vi "DriveModuleControl_TravTunePID.vi"(8 "error in":errorcluster, 9 "Actual State":T1={"Speed"=0.0, "Angle"={"VALUE"=0.0, "COS"=1.0, "SIN"=0.0}} {"Angle"."SIN" format="%13.4f"; "Angle"."COS" format="%13.4f"; "Angle"."VALUE" format="%13.4f"}, 10 "Desired State":T1={"Speed"=0.0, "Angle"={"VALUE"=0.0, "COS"=1.0, "SIN"=0.0}} {"Angle"."SIN" format="%13.4f"; "Angle"."COS" format="%13.4f"; "Angle"."VALUE" format="%13.4f"}, 11 "ModualNamePrefix":i32) -> (0 "error out":errorcluster)   [LabVIEW 2023]
uses:
  <vilib>/Rock Robotics/WPI/ThirdParty/JAS_Junk/TrajLib/TypeDef/SWERVE_DRIVE_MODULE_STATE.ctl
  <vilib>/Rock Robotics/WPI/ThirdParty/JAS_Junk/TrajLib/TypeDef/ROTATION2D.ctl
  <vilib>/Rock Robotics/WPI/ThirdParty/REV Robotics/REVLib/Typedef/Spark MAX Control Type.ctl
  <vilib>/Rock Robotics/WPI/ThirdParty/JAS_Junk/TrajLib/Rotation2d_Minus.vi
  <vilib>/Rock Robotics/WPI/ThirdParty/JAS_Junk/TrajLib/Rotation2d_GetRadians.vi
  <vilib>/Rock Robotics/WPI/ThirdParty/JAS_Junk/TrajLib/SwerveModuleState_New.vi
  <vilib>/Rock Robotics/WPI/ThirdParty/JAS_Junk/TrajLib/Rotation2d_RotateBy.vi
  <vilib>/Rock Robotics/WPI/ThirdParty/JAS_Junk/TrajLib/Rotation2d_CreateAngle.vi
  <vilib>/Rock Robotics/WPI/ThirdParty/JAS_Junk/TrajLib/SimpleMotorFF_Calculate.vi
  <vilib>/Rock Robotics/WPI/ThirdParty/JAS_Junk/TrajLib/PIDController_AtSetpoint.vi
  <vilib>/Rock Robotics/WPI/ThirdParty/JAS_Junk/TrajLib/PIDController_SetPIDF.vi
  <vilib>/Rock Robotics/WPI/ThirdParty/JAS_Junk/TrajLib/PIDController_SetDerivativeFilter.vi
  <vilib>/Rock Robotics/WPI/ThirdParty/JAS_Junk/TrajLib/PIDController_SetIntegratorRange.vi
  <vilib>/Rock Robotics/WPI/ThirdParty/JAS_Junk/TrajLib/PIDController_SetTolerancePandV.vi
  <vilib>/Rock Robotics/WPI/ThirdParty/JAS_Junk/TrajLib/PIDController_DisableContinousInput.vi
  <vilib>/Rock Robotics/WPI/ThirdParty/JAS_Junk/TrajLib/PIDController_EnableContinousInput.vi
  <vilib>/Rock Robotics/WPI/ThirdParty/JAS_Junk/TrajLib/PIDController_Reset.vi
  <vilib>/Rock Robotics/WPI/ThirdParty/JAS_Junk/TrajLib/PIDController_New.vi
  <vilib>/Rock Robotics/WPI/ThirdParty/JAS_Junk/TrajLib/PIDController_SetOutputLimits.vi
  <vilib>/Rock Robotics/WPI/ThirdParty/JAS_Junk/TrajLib/VI/PIDController_SetIntegratorZone.vi
  <vilib>/Rock Robotics/WPI/ThirdParty/JAS_Junk/TrajLib/Timer_New.vi
  <vilib>/Rock Robotics/WPI/ThirdParty/JAS_Junk/TrajLib/Rotation2d_UnaryMinus.vi
  <vilib>/Rock Robotics/WPI/ThirdParty/JAS_Junk/TrajLib/Rotation2d_CreateXY.vi
  <vilib>/Rock Robotics/WPI/ThirdParty/JAS_Junk/TrajLib/PIDController_NewPeriod.vi
  <vilib>/Rock Robotics/WPI/ThirdParty/JAS_Junk/TrajLib/Util_CalcDist.vi
  <vilib>/Rock Robotics/SystemInterfaces/NetworkCommunication/NetComm_UsageReport_report.vi
  DriveGlobal.vi
  <vilib>/Utility/semaphor.llb/Obtain Semaphore Reference.vi
  <vilib>/Rock Robotics/WPI/ThirdParty/JAS_Junk/TrajLib/Timer_Reset.vi
  <vilib>/Rock Robotics/WPI/ThirdParty/JAS_Junk/TrajLib/Timer_Start.vi
  <vilib>/Rock Robotics/WPI/ThirdParty/JAS_Junk/TrajLib/Timer_Stop.vi
  <vilib>/Rock Robotics/WPI/ThirdParty/JAS_Junk/TrajLib/Timer_HasPeriodPassedOnce.vi
  <vilib>/Rock Robotics/WPI/ThirdParty/Phoenix6/Phoenix6_Device_RefNumRegistryGet.vi
  <vilib>/Rock Robotics/WPI/MotorControl/WPI_MotorControlRefNum Registry Get.vi
  <vilib>/Rock Robotics/WPI/ThirdParty/JAS_Junk/TrajLib/Globals/Util_LibraryGlobals.vi
  <vilib>/Rock Robotics/WPI/ThirdParty/JAS_Junk/TrajLib/PIDController_AdvCalculate_FF_Sp_Pv.vi
  DriveTuningGlobals.vi
  <vilib>/Rock Robotics/WPI/ThirdParty/JAS_Junk/TrajLib/Trajectory_Library.lvlib
panel:
  out "TravelMotorDmd":dbl
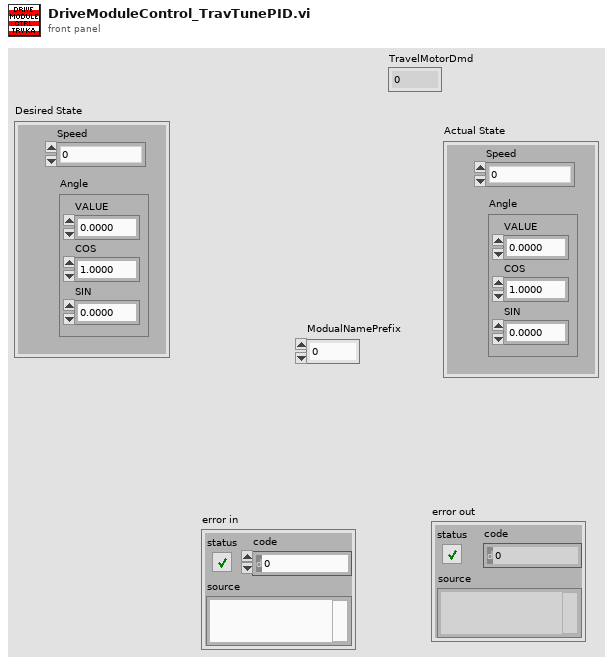
[diagram p1: front panel]
types:
  T1 = typedef "Trajectory_Library.lvlib/SWERVE_DRIVE_MODULE_STATE.ctl" = cluster{"Speed":dbl, "Angle":T2}
  T2 = typedef "Trajectory_Library.lvlib/ROTATION2D.ctl" = cluster{"VALUE":dbl, "COS":dbl, "SIN":dbl}
  T3 = typedef "Spark MAX Control Type.ctl" = enum16{"Percent VBus", "Voltage", "Velocity", "Position", "Smart Motion", "Current", "Smart Velocity", "MAXMotion Position", "MAXMotion Velocity"}
  T4 = enum16{"Ziegler Nicols - Fast", "Ziegler Nicols - Normal", "Ziegler Nicols - Slow", "CHR regulator - 0% overshoot", "CHR regulator - 20% overshoot", "CHR servo - 0 % overshoot", "CHR servo - 20% overshoot"}
  T5 = typedef "WPI_MotorControlDeviceRef.ctl" = cluster{"DeviceStatus":errorcluster, "Type":T6, "PWM":cluster{"PWM Channel":T7, "DeadBand":T8}, "CAN":cluster{"Device Number":u8, "SetOutput VI Ref":variant, "GetOutput VI Ref":variant, "Enable VI Ref":variant, "Disable VI Ref":variant, "Data":variant}, "Invert":bool, "DIO PWM":cluster{"PWM \"Enable\" Channel":T7, "DIOChannel":T9, "PWM Rate":dbl}}
  T6 = typedef "WPI_MotorControlType.ctl" = enum16{"PWM", "CAN", "DIO PWM"}
  T7 = typedef "FPGA_DIOPWMChannel.ctl" = enum8{"PWM 0", "PWM 1", "PWM 2", "PWM 3", "PWM 4", "PWM 5", "PWM 6", "PWM 7", "PWM 8", "PWM 9", "PWM MXP 0", "PWM MXP 1", "PWM MXP 2", "PWM MXP 3", "PWM MXP 4", "PWM MXP 5", "PWM MXP 6", "PWM MXP 7", "PWM MXP 8", "PWM MXP 9", "Invalid"}
  T8 = typedef "WPI_PWMDeadband.ctl" = cluster{"Name":string, "maxPositivePwm":i32, "minPositivePwm":i32, "centerPwm":i32, "maxNegativePwm":i32, "minNegativePwm":i32, "angularRange":u16}
  T9 = typedef "FPGA_DIOChannel.ctl" = enum8{"DIO 0", "DIO 1", "DIO 2", "DIO 3", "DIO 4", "DIO 5", "DIO 6", "DIO 7", "DIO 8", "DIO 9", "DIO MXP 0", "DIO MXP 1", "DIO MXP 2", "DIO MXP 3", "DIO MXP 4", "DIO MXP 5", "DIO MXP 6", "DIO MXP 7", "DIO MXP 8", "DIO MXP 9", "DIO MXP 10", "DIO MXP 11", "DIO MXP 12", "DIO MXP 13", "DIO MXP 14", "DIO MXP 15", "SPI Port CS1", "SPI Port CS2", "SPI Port CS3", "SPI Port MISO", "SPI Port MOSI", "Invalid"}
  T10 = typedef "Trajectory_Library.lvlib/SIMPLE_MOTOR_FF.ctl" = cluster{"Ks":dbl, "Kv":dbl, "Ka":dbl, "KnInv":dbl}
  T11 = typedef "Trajectory_Library.lvlib/PID_ADV_LIMITS.ctl" = cluster{"MaxInput":dbl, "MinInput":dbl, "Continuous":bool, "MaxOutput":dbl, "MinOutput":dbl}
  T12 = typedef "Trajectory_Library.lvlib/PID_ADV_TUNING.ctl" = cluster{"Kf":dbl, "Kp":dbl, "Ki":dbl, "Kd":dbl, "MaximumIntegral":dbl, "MinimumIntegral":dbl, "Filter Derivative":bool, "IntegralZone":dbl}
  T13 = cluster{"Controller Constant Type":enum16{"Ziegler Nicols - Fast", "Ziegler Nicols - Normal", "Ziegler Nicols - Slow", "CHR regulator - 0% overshoot", "CHR regulator - 20% overshoot", "CHR servo - 0 % overshoot", "CHR servo - 20% overshoot"}, "Type of Controller":enum16{"P", "PI", "PID"}, "CO Offset":dbl, "Kn":dbl, "Tuning Tolerance":dbl, "Plant Tolerance":dbl, "Newest Avg Time ":i32, "Long Ave Time":i32}
  T14 = cluster{"Plant Gain (K)":dbl, "Time Constant (T)":dbl, "Dead Time (L)":dbl, "stimulus operating point":dbl, "response operating point":dbl}
  T15 = cluster{"proportional gain (Kp)":dbl, "integral time (Ki / Sec)":dbl, "derivative time (Kd /Sec)":dbl}
  T16 = cluster{"Const Done":bool, "Plant Done":bool, "PV Std Dev":dbl, "CO Std Dev":dbl}
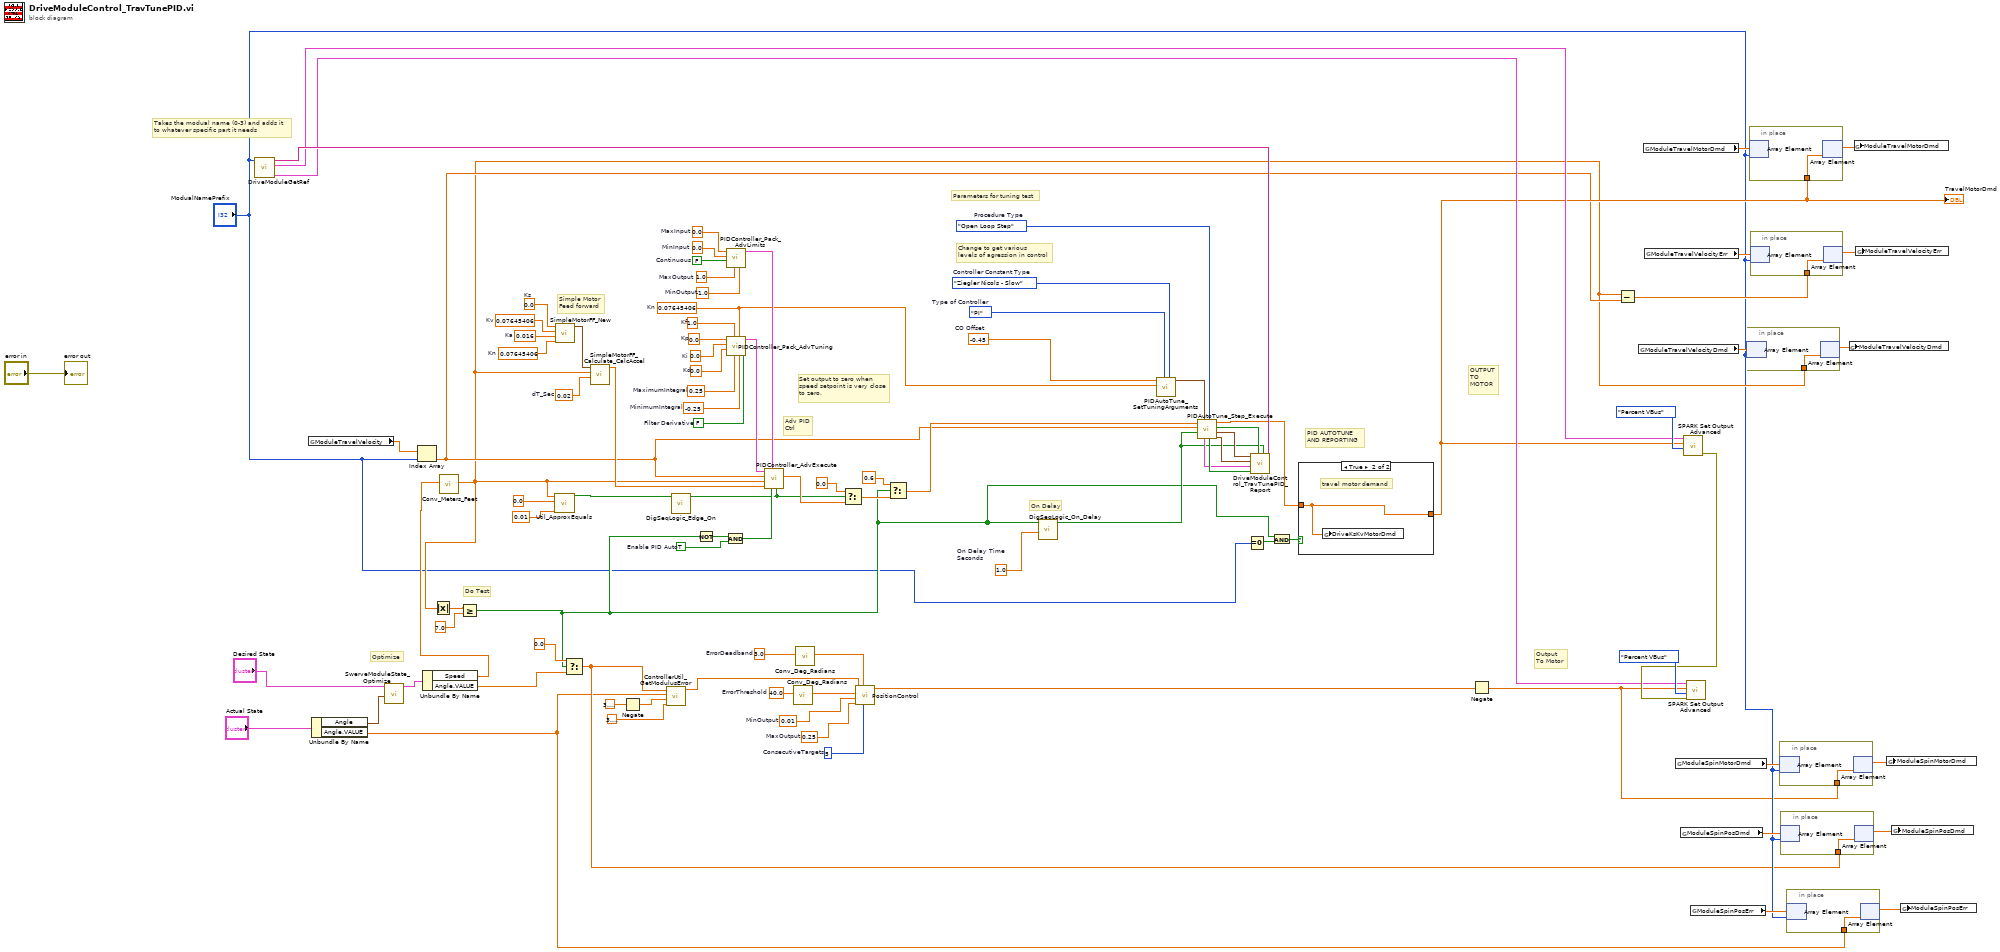
[diagram p0: block diagram]
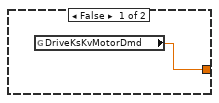
[diagram p2: hidden frame]
diagram:
  w33 = 1.0  # On Delay Time Seconds
  w44 = enum16{"Open Loop Step", "Closed Loop Step"}."Open Loop Step"  # Procedure Type
  w45 = T4."Ziegler Nicols - Slow"  # Controller Constant Type
  w46 = enum16{"P", "PI", "PID"}."PI"  # Type of Controller
  w47 = -0.45  # CO Offset
  w56 = TRUE  # Enable PID Auto
  w43 = 0.07645406  # Kn
  w76 = 0.0  # Kp
  w75 = 0.0  # Ki
  w74 = 0.0  # Kd
  w73 = 1.0  # Kf
  w72 = 0.25  # MaximumIntegral
  w71 = -0.25  # MinimumIntegral
  w70 = FALSE  # Filter Derivative
  w68 = 0.0  # MinInput
  w67 = FALSE  # Continuous
  w66 = 1.0  # MaxOutput
  w69 = -1.0  # MinOutput
  w65 = 0.0  # MaxInput
  w82 = 0.07645406  # Kn
  w81 = 0.02  # dT_Sec
  w79 = 0.0  # Ks
  w78 = 0.07645406  # Kv
  w77 = 0.016  # Ka
  w90 = 5  # ConsecutiveTargets
  w88 = 0.25  # MaxOutput
  w91 = 0.01  # MinOutput
  w85 = 40.0  # ErrorThreshold
  w87 = 3.0  # ErrorDeadband
  # "On Delay"
  # "Output\nTo Motor"
  # "OUTPUT\nTO \nMOTOR"
  # "PID AUTOTUNE\nAND REPORTING"
  # "Change to get various\nlevels of agression in control"
  # "Parameters for tuning test"
  # "Do Test"
  # "Optimize"
  # "Set output to zero when\nspeed setpoint is very close\nto zero."
  # "Adv PID\nCtrl"
  # "Simple Motor\nFeed forward"
  # "Takes the modual name (0-3) and adds it \nto whatever specific part it needs"
  n1 = call "DriveModuleGetRef.vi"("ModualNamePrefix"="ModualNamePrefix") -> ("SpinMot"=w21:T5, "TravMot"=w22:T5, "TravStr"=w39:string)  [unwired: 5 in, 3 out]
  n2 = global read "DriveGlobal.vi" "ModuleTravelVelocity"() -> (w61:dbl[])
  n3 = Unbundle By Name("Actual State") -> ("Angle"=w96:T2, "Angle.VALUE"=w1:dbl)
  n4 = call <vilib>:"SwerveModuleState_Optimize.vi"("CurrentAngle"=w96, "Desired State"="Desired State") -> ("out SWERVE_DRIVE_MODULE_STATE"=w94:T1)  [unwired: 9 in]
  n5 = Index Array(array=w61, index="ModualNamePrefix") -> (element=w12:dbl)
  n6 = Unbundle By Name(w94) -> ("Speed"=w53:dbl, "Angle.VALUE"=w50:dbl)
  n7 = call <vilib>:"Conv_Meters_Feet.vi"("Meters"=w53) -> ("Feet"=w11:dbl)  [unwired: 10 in]
  n8 = Absolute Value(x=w11) -> (abs(x)=w52:dbl)
  n9 = Greater Or Equal?(x=w52, y=7.0) -> (x >= y?=w28:bool)
  n10 = call <vilib>:"Util_ApproxEquals.vi"("Tolerance"=0.01, "Value 2"=0.0, "Value 1"=w11) -> ("ApproxEquals"=w27:bool)  [unwired: 8 in]
  n11 = call <vilib>:"SimpleMotorFF_New.vi"("Kn"=w82, "Ka"=w77, "Kv"=w78, "Ks"=w79) -> ("SIMPLE_MOTOR_FF"=w80:T10)  [unwired: 7 in]
  n12 = Select(t=0.0, s=w28, f=w50) -> (s? t:f=w2:dbl)
  n13 = call <vilib>:"SimpleMotorFF_Calculate_CalcAccel.vi"("dT_Sec"=w81, "VelSp"=w11, "SIMPLE_MOTOR_FF"=w80) -> ("FeedForward"=w62:dbl)  [unwired: 8 in]
  n14 = Negate(x=3.141592653589793) -> (-x=w95:dbl)
  n15 = call <vilib>:"ControllerUtil_GetModulusError.vi"("Maximum_Input"=3.141592653589793, "Minimum_Input"=w95, "Measurerment(PV)"=w1, "Reference(SP)"=w2) -> ("Error"=w89:dbl)  [unwired: 7 in]
  n16 = call <vilib>:"DigSeqLogic_Edge_On.vi"("Input"=w27) -> ("On Edge"=w26:bool)  [unwired: 10 in]
  n17 = Not(x=w28) -> (.not. x?=w57:bool)
  n18 = And(x=w57, y=w56) -> (x .and. y?=w58:bool)
  n19 = call <vilib>:"PIDController_Pack_AdvLimits.vi"("MinOutput"=w69, "MaxOutput"=w66, "Continuous"=w67, "MinInput"=w68, "MaxInput"=w65) -> ("Adv PID Limits"=w63:T11)  [unwired: 6 in]
  n20 = call <vilib>:"PIDController_Pack_AdvTuning.vi"("Filter Derivative"=w70, "MinimumIntegral"=w71, "Kn"=w43, "MaximumIntegral"=w72, "Kf"=w73, "Kd"=w74, "Ki"=w75, "Kp"=w76) -> ("Adv PID Tuning"=w64:T12)  [unwired: 3 in]
  n21 = call <vilib>:"PIDController_AdvExecute.vi"("Reset"=w26, "Auto"=w58, "Adv PID Limits"=w63, "FF-FeedForward"=w62, "SP-SetPoint"=w11, "PV-Measurement"=w12, "Adv PID Tuning"=w64) -> ("CO-ControlOutput"=w55:dbl)  [unwired: 2 in, 2 out]
  n22 = call <vilib>:"Conv_Deg_Radians.vi"("Degress"=w85) -> ("Radians"=w84:dbl)  [unwired: 10 in]
  n23 = call <vilib>:"Conv_Deg_Radians.vi"("Degress"=w87) -> ("Radians"=w86:dbl)  [unwired: 10 in]
  n24 = Select(t=0.0, s=w26, f=w55) -> (s? t:f=w36:dbl)
  n25 = call "PositionControl.vi"("ConsecutiveTargets"=w90, "ErrorDeadband"=w86, "MaxOutput"=w88, "MinOutput"=w91, "ErrorThreshold"=w84, "Error"=w89) -> ("OutputValue"=w83:dbl)  [unwired: 3 in, 2 out]
  n26 = Select(t=0.6, s=w28, f=w36) -> (s? t:f=w35:dbl)
  n27 = call <vilib>:"DigSeqLogic_On_Delay.vi"("Delay"=w33, "Input"=w28) -> ("Output"=w32:bool)  [unwired: 8 in, 1 out]
  n28 = call <vilib>:"PIDAutoTune_SetTuningArguments.vi"("Controller Constant Type"=w45, "Type of Controller"=w46, "Kn"=w43, "CO Offset"=w47) -> ("Configuration Parameters"=w48:T13)  [unwired: 7 in]
  n29 = call <vilib>:"PIDAutoTune_Step_Execute.vi"("Procedure Type"=w44, "Configuration Parameters"=w48, "Tune"=w32, "Measurement  (PV)"=w12, "Control Output (Co)"=w35) -> ("Plant and Test Data"=w41:T14, "New Tuning Parameters"=w42:T15, "Tuning Done"=w40:bool, "Adj CO"=w31:dbl, "Error Occured"=w38:bool, "Diagnostic Info"=w37:T16)  [unwired: 1 in]
  n30 = Equal To 0?(x="ModualNamePrefix") -> (x = 0?=w29:bool)
  n31 = call "DriveModuleControl_TravTunePID_Report.vi"("Network Table Prefix"=w39, "TestInProgress"=w32, "Tuning Done"=w40, "Error Occured"=w38, "Diagnostic Info"=w37, "Plant and Test Data"=w41, "New Tuning Parameters"=w42) -> ()  [unwired: 5 in]
  n32 = And(x=w28, y=w29) -> (x .and. y?=w30:bool)
  n33 = case shown="True" w30 {
    tunnel: [w100 w101] -> w13
    tunnel: w31 -> [_ w101]
    frame False {
      n34 = global read "DriveTuningGlobals.vi" "DriveKsKvMotorDmd"() -> (w100:dbl)
    }
    frame True {
      # "travel motor demand"
      n35 = global write "DriveTuningGlobals.vi" "DriveKsKvMotorDmd"(w101) -> ()
    }
  }
  "TravelMotorDmd" <- w13
  n36 = Negate(x=w83) -> (-x=w3:dbl)
  n37 = Subtract(x=w11, y=w12) -> (x-y=w18:dbl)
  n38 = global read "DriveGlobal.vi" "ModuleTravelVelocityDmd"() -> (w19:dbl[])
  n39 = global read "DriveGlobal.vi" "ModuleTravelMotorDmd"() -> (w14:dbl[])
  n40 = global read "DriveGlobal.vi" "ModuleTravelVelocityErr"() -> (w16:dbl[])
  n41 = global read "DriveGlobal.vi" "ModuleSpinMotorDmd"() -> (w9:dbl[])
  n42 = global read "DriveGlobal.vi" "ModuleSpinPosDmd"() -> (w7:dbl[])
  n43 = call <vilib>:"SPARK Set Output Advanced.vi"("Control Mode"=Spark_MAX_Control_Type."Percent VBus", "Setpoint"=w13, "MotorControlDevRef"=w22) -> ("error out"=w23:errorcluster)  [unwired: 7 in, 1 out]
  n44 = call <vilib>:"SPARK Set Output Advanced.vi"("error in (no error)"=w23, "Control Mode"=Spark_MAX_Control_Type."Percent VBus", "Setpoint"=w3, "MotorControlDevRef"=w21) -> ()  [unwired: 6 in, 2 out]
  n45 = global read "DriveGlobal.vi" "ModuleSpinPosErr"() -> (w5:dbl[])
  n46 = in-place {
    in-place-border: w11 -> [w102]
    n47 = in-place-array #1(w19, "ModualNamePrefix") -> ()  [unwired: 1 out]
    n48 = in-place-array #1(w102) -> (w20:dbl[])  [unwired: 1 out]
  }
  n49 = in-place {
    in-place-border: w13 -> [w103]
    n50 = in-place-array #2(w14, "ModualNamePrefix") -> ()  [unwired: 1 out]
    n51 = in-place-array #2(w103) -> (w15:dbl[])  [unwired: 1 out]
  }
  n52 = in-place {
    in-place-border: w18 -> [w104]
    n53 = in-place-array #3(w16, "ModualNamePrefix") -> ()  [unwired: 1 out]
    n54 = in-place-array #3(w104) -> (w17:dbl[])  [unwired: 1 out]
  }
  n55 = in-place {
    in-place-border: w3 -> [w105]
    n56 = in-place-array #4(w9, "ModualNamePrefix") -> ()  [unwired: 1 out]
    n57 = in-place-array #4(w105) -> (w10:dbl[])  [unwired: 1 out]
  }
  n58 = in-place {
    in-place-border: w2 -> [w106]
    n59 = in-place-array #5(w7, "ModualNamePrefix") -> ()  [unwired: 1 out]
    n60 = in-place-array #5(w106) -> (w8:dbl[])  [unwired: 1 out]
  }
  n61 = in-place {
    in-place-border: w1 -> [w107]
    n62 = in-place-array #6(w5, "ModualNamePrefix") -> ()  [unwired: 1 out]
    n63 = in-place-array #6(w107) -> (w6:dbl[])  [unwired: 1 out]
  }
  n64 = global write "DriveGlobal.vi" "ModuleTravelVelocityDmd"(w20) -> ()
  n65 = global write "DriveGlobal.vi" "ModuleTravelMotorDmd"(w15) -> ()
  n66 = global write "DriveGlobal.vi" "ModuleTravelVelocityErr"(w17) -> ()
  n67 = global write "DriveGlobal.vi" "ModuleSpinMotorDmd"(w10) -> ()
  n68 = global write "DriveGlobal.vi" "ModuleSpinPosDmd"(w8) -> ()
  n69 = global write "DriveGlobal.vi" "ModuleSpinPosErr"(w6) -> ()
  "error out" <- "error in"
